vi "ReadTemp_avg.vi"() -> ()   [LabVIEW 2010]
uses:
  <vilib>/Analysis/NI_AALBase.lvlib
panel:
  out "Progress":u8(slide) scale=0.0..100.0
  out "Temp. Error (°C)":dbl
  out "Temp. Average (°C)":dbl
  in  "mode (0)":i16
  in  "error in":errorcluster
  in  "address string":string="19"
  out "error out":errorcluster
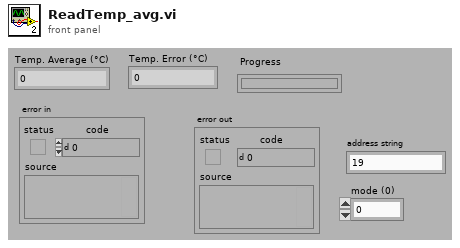
[diagram p1: front panel]
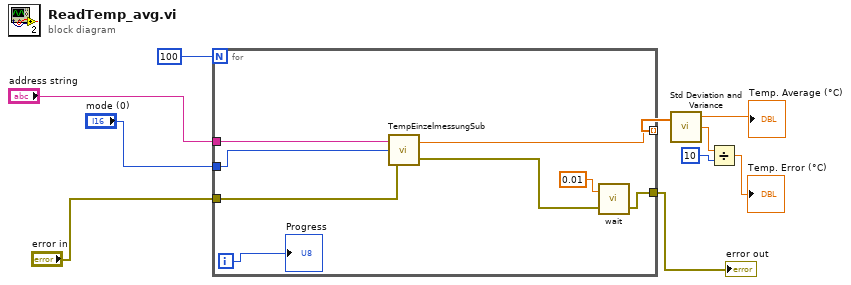
[diagram p0: block diagram]
diagram:
  n1 = for {
    N: 100 -> [_]
    tunnel: "mode (0)" -> [w17]
    tunnel: "address string" -> [w18]
    tunnel: "error in" -> [w16]
    tunnel: [w15] -> w6 mode=indexing
    tunnel: [w12] -> w1
    i -> [w14]
    n2 = call "TempEinzelmessungSub.vi"("error in"=w16, "mode (0)"=w17, "address string"=w18) -> ("error out"=w13:errorcluster, "Numeric"=w15:dbl)
    n3 = call "wait.vi"("error in"=w13, "Wartezeit in Sek"=0.01) -> ("error out"=w12:errorcluster)  [unwired: 1 in]
    "Progress" <- w14
  }
  "error out" <- w1
  n4 = call <vilib>:"Std Deviation and Variance.vi"("X"=w6) -> ("mean"=→"Temp. Average (°C)":dbl, "standard deviation"=w3:dbl)  [unwired: 1 in, 1 out]
  n5 = Divide(x=w3, y=10) -> (x/y=→"Temp. Error (°C)":dbl)
